vi "FPGA Main.vi"() -> ()   [LabVIEW 2014]
uses:
  <vilib>/Platform/TimedLoop/XDataNode/timing_clust.ctl
  <vilib>/Platform/TimedLoop/XDataNode/nitl_modes.ctl
  <vilib>/Platform/TimedLoop/XDataNode/wakeup.ctl
  <vilib>/rvi/eio/common/nirviEmuClasses.ctl
  <vilib>/rvi/Emulation/niFpgaGetClockAttributes.vi
  <vilib>/rvi/Emulation/niFpgaSctlEmulationGetInTimedLoop.vi
  <vilib>/rvi/Emulation/niFpgaEmulationReportErrorSimple.vi
  FPGA/VIs/FPGA Globals.vi
  <vilib>/rvi/Emulation/niFpgaProcessEmulError.vi
  <vilib>/rvi/eio/common/nirviEmuTemplateMethod_errors.vi
  <vilib>/rvi/Emulation/niFpgaCriticalErrorInLSC.vi
  <vilib>/rvi/interface/RandomDataEmulation/niFpgaRandomDataHandleErrors.vi
  <vilib>/eio/EIONode/EIONode.xnode
  <vilib>/eio/EIOGrowableMethodNode/genericMethod/EIOGrowableMethodNode.xnode
  <vilib>/rvi/eio/nirviEIOMethodImplementation/nirviEIOMethodImplementation.xnode
  <vilib>/rvi/eio/nirviErrorMerge/nirviErrorMerge.xnode
  <vilib>/rvi/DataTransferAndStorage/Container/XNode/niFpgaContainer.xnode
  <vilib>/rvi/interface/RandomDataEmulation/nirviRandomDataFpgaReadWriteTemplate.vi
  <vilib>/Platform/TimedLoop/XDataNode/XDataNode.xnode
  <vilib>/Platform/TimedLoop/XDataNode/XDNodeRunTimeDep.lvlib
panel:
  out "ADC First  Sample Recieved":bool
  out "Interlock HB":bool
  out "Global Triggered":bool
  in  "ADC Mask":bool[](array[boolean])=[FALSE, FALSE, FALSE, FALSE, FALSE, FALSE, FALSE, FALSE, FALSE, FALSE, FALSE, FALSE, FALSE, FALSE, FALSE, FALSE]
  out "DIN":bool[](array[boolean])
  out "ADC Triggered":bool
  out "DIN Triggered":bool
  out "ADC Min Threshold Triggered":bool[](array[boolean])
  out "ADC Max Threshold Triggered":bool[](array[boolean])
  in  "ADC Threshold max value":sgl[](array[numeric])=[0.0, 0.0, 0.0, 0.0, 0.0, 0.0, 0.0, 0.0, 0.0, 0.0, 0.0, 0.0, 0.0, 0.0, 0.0, 0.0]
  in  "ADC Threshold min value":sgl[](array[numeric])=[0.0, 0.0, 0.0, 0.0, 0.0, 0.0, 0.0, 0.0, 0.0, 0.0, 0.0, 0.0, 0.0, 0.0, 0.0, 0.0]
  out "Current sample":sgl[](array[numeric])
  out "ADC Sampling Timeout":bool
  out "Different Channel Count":bool
  out "Actual Loop Period (ticks)":u32
  in  "Interlock on":bool
  in  "Number of Channels":i16
  out "Data Acq Running":bool
  in  "Data Acq Stop":bool
  in  "External trigger":bool
  in  "Number samples\nafter trigger":i32
  in  "DIN Mask":bool[](array[boolean])=[FALSE, FALSE, FALSE, FALSE, FALSE, FALSE, FALSE, FALSE]
  in  "Sample Period (uSec)":u32=10
  out "Overwrite":bool
  out "Sample Gated":bool
  out "Error":bool
  out "FPGA Error":errorcluster
  out "DMA FIFO Full":bool
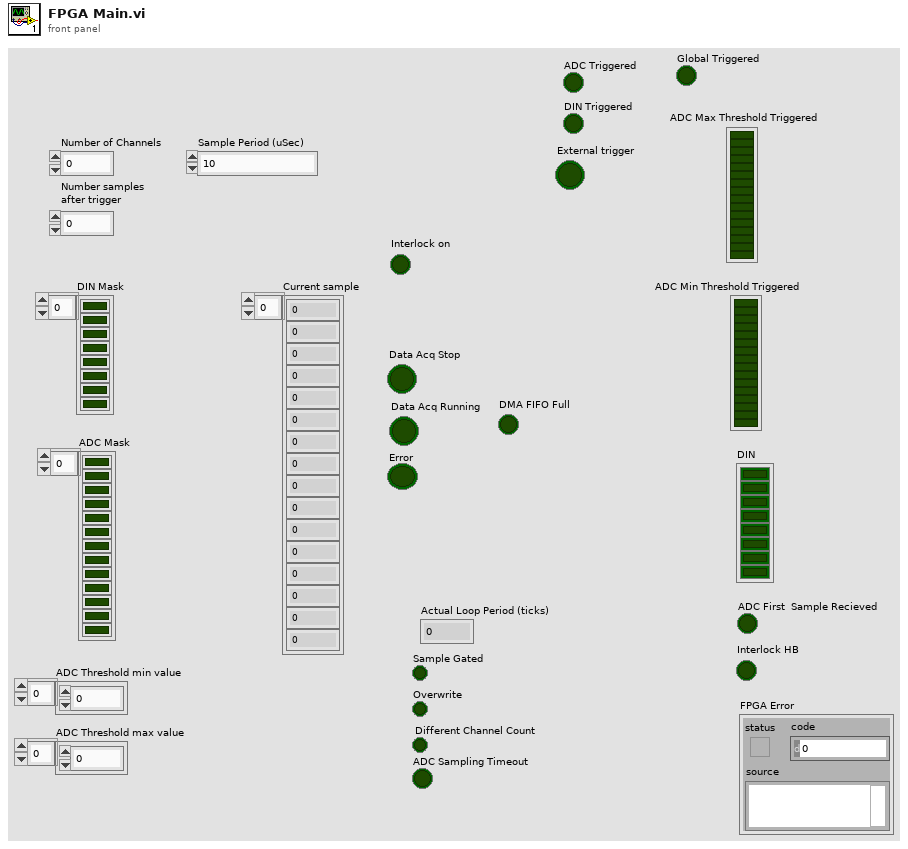
[diagram p1: front panel]
types:
  T1 = typedef "nirviEmuClasses.ctl" = enum16{"IO Read", "IO Write", "Method", "Property Read", "Property Write"}
  T2 = typedef "XDNodeRunTimeDep.lvlib/timing_clust.ctl" = cluster{"Expected End [f-1]":u64, "Actual End [f-1]":u64, "Finished Late? [f-1]":bool, "Expected End [i-1]":u64, "Actual End [i-1]":u64, "Finished Late? [i-1]":bool, "Expected Start [i]":u64, "Actual Start [i]":u64, "Expected Start [f]":u64, "Actual Start [f]":u64, "Source Name":string, "Structure Name":string, "Period":i64, "Deadline":i64, "Offset":i64, "Start":i64, "Priority":i32, "Timeout":i32, "Mode":T3, "Wakeup Reason":T4, "Error":errorcluster, "Source Type":string, "Secondary Source Type":string, "Global End Time":u64, "Global Start Time":u64, "Frame Duration":u64, "Iteration Duration":u64, "Assigned CPU":i32, "I/O Scan Engine Mode":u32}
  T3 = typedef "XDNodeRunTimeDep.lvlib/nitl_modes.ctl" = enum32{"No Change", "Process missed periods, maintain original phase", "Discard missed periods, maintain original phase", "Process missed periods, ignore original phase", "Discard missed periods, ignore original phase"}
  T4 = typedef "XDNodeRunTimeDep.lvlib/wakeup.ctl" = enum32{"Normal", "Aborted", "Asynchronous wakeup", "Timing source error", "Timed loop error", "Timeout"}
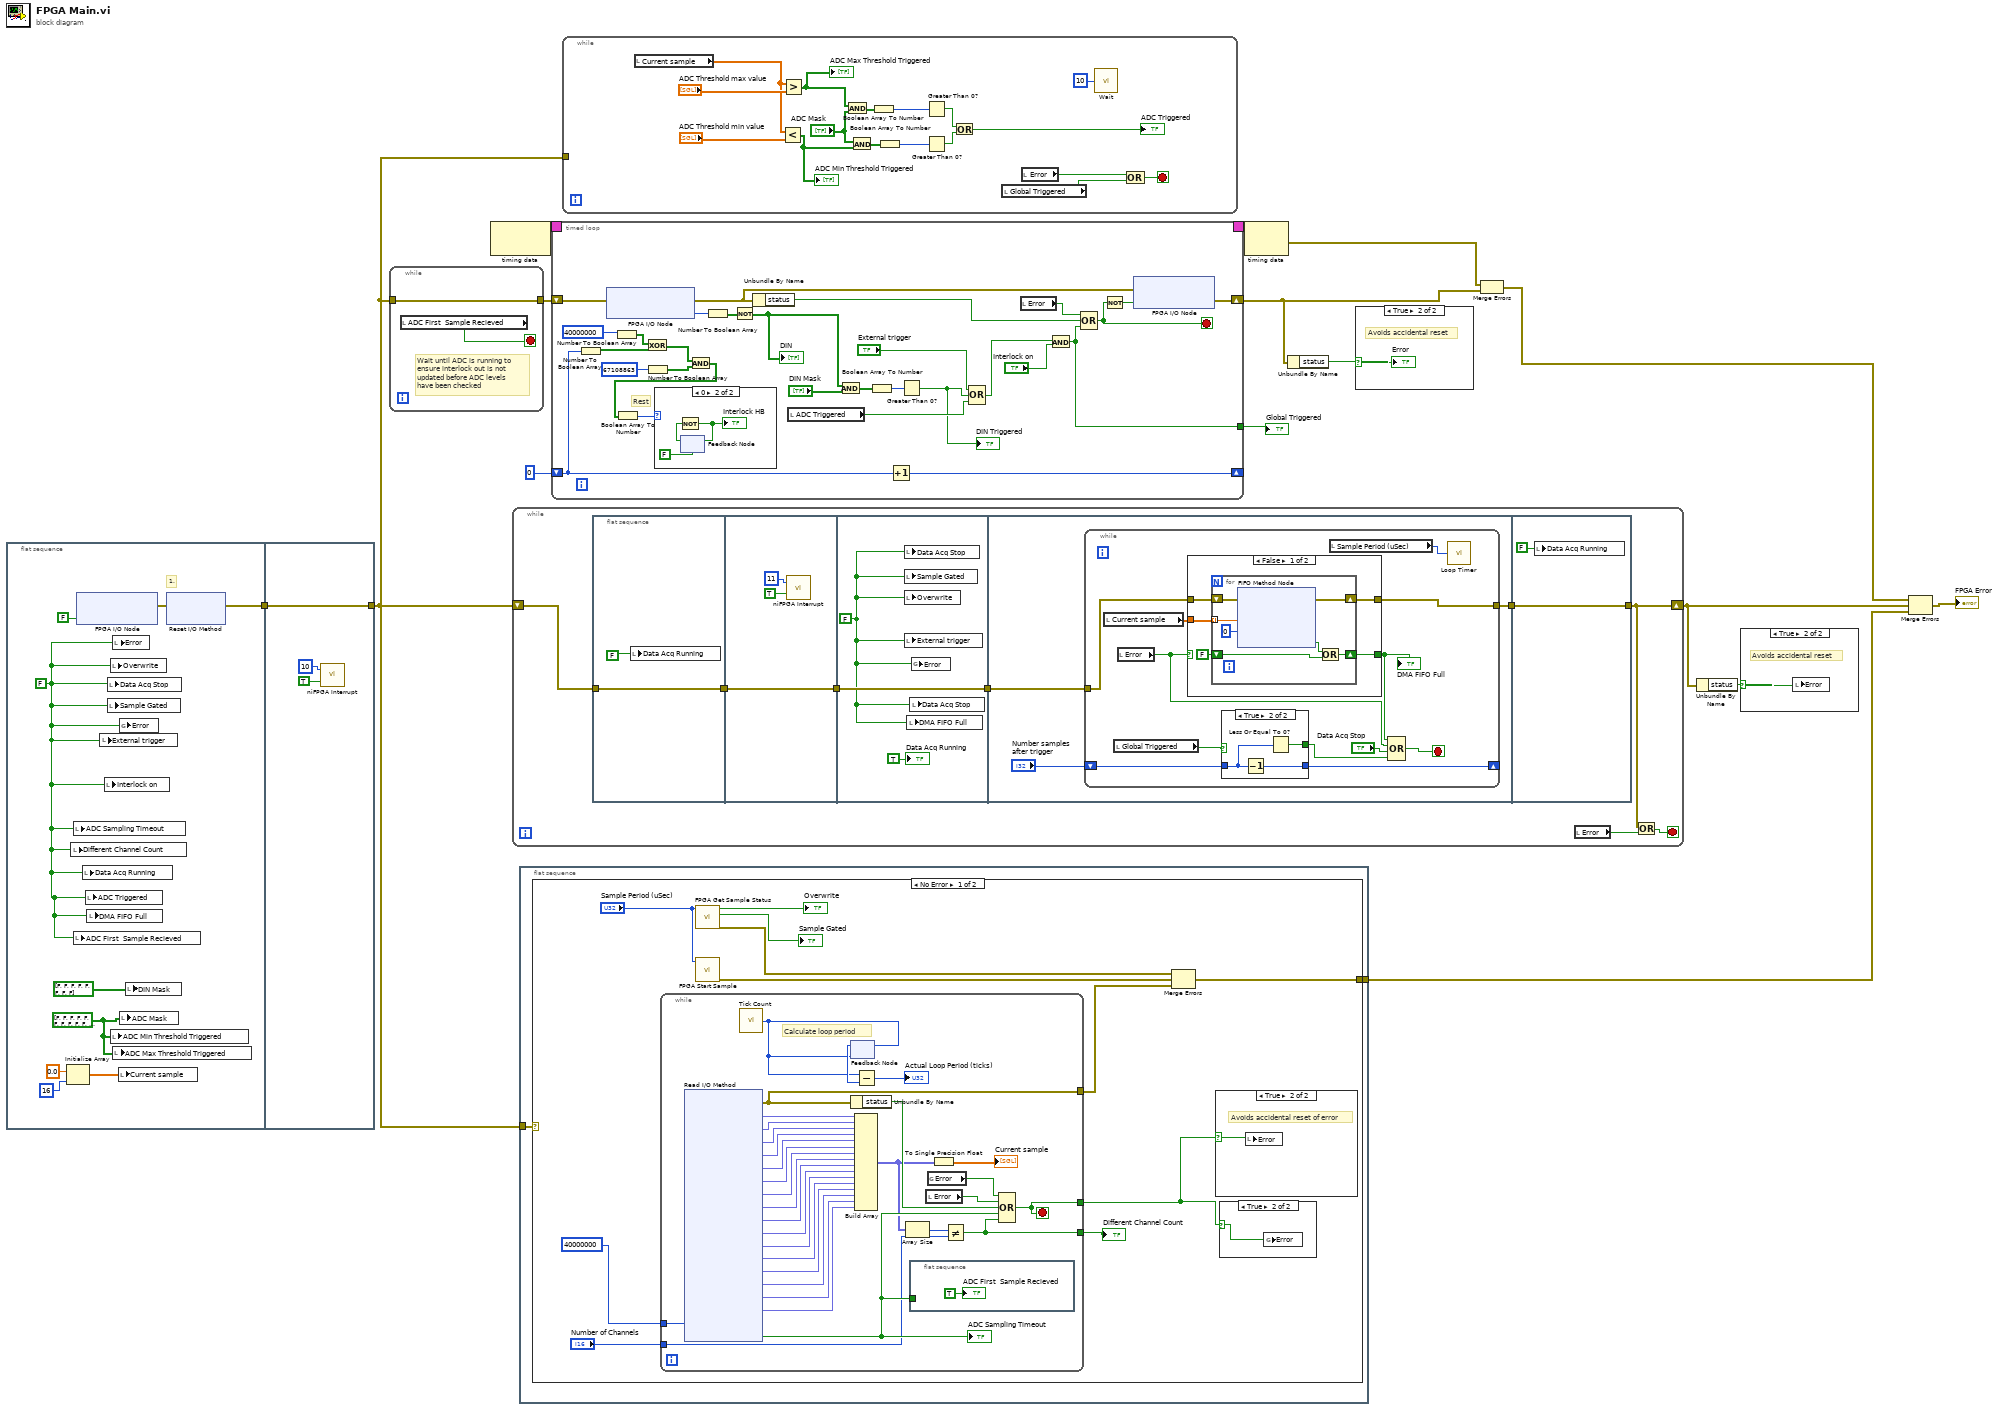
[diagram p0: block diagram]
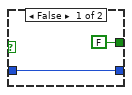
[diagram p8: hidden frame]
diagram:
  n1 = flat-sequence {
    tunnel: [w24] -> w11
    tunnel: [w71] -> w1
    tunnel: w11 -> [w71]
    frame #0 {
      w17 = bool[] [FALSE, FALSE, FALSE, FALSE, FALSE, FALSE, FALSE, FALSE, FALSE, FALSE, FALSE, FALSE, FALSE, FALSE, FALSE, FALSE] ("Mask")
      w16 = FALSE ("Stopped")
      # "1."
      n2 = Initialize Array(sgl 0.0 ("element"), 16 ("dimension size")) -> (w19:sgl[])
      n3 = local write "Different Channel Count"(w16) -> ()
      n4 = local write "ADC Sampling Timeout"(w16) -> ()
      n5 = local write "ADC First  Sample Recieved"(w16) -> ()
      n6 = xnode "FPGA I/O Node"("Mod1/DIO0"=FALSE) -> ("error out"=w23:errorcluster)  [unwired: 2 in, 1 out]
      n7 = local write "Data Acq Running"(w16) -> ()
      n8 = local write "ADC Triggered"(w16) -> ()
      n9 = local write "DMA FIFO Full"(w16) -> ()
      n10 = local write "External trigger"(w16) -> ()
      n11 = local write "Interlock on"(w16) -> ()
      n12 = local write "Data Acq Stop"(w16) -> ()
      n13 = local write "Sample Gated"(w16) -> ()
      n14 = local write "Overwrite"(w16) -> ()
      n15 = local write "ADC Min Threshold Triggered"(w17) -> ()
      n16 = local write "Error"(w16) -> ()
      n17 = local write "ADC Max Threshold Triggered"(w17) -> ()
      n18 = local write "Current sample"(w19) -> ()
      n19 = global write "FPGA Globals.vi" "Error"(w16) -> ()
      n20 = local write "ADC Mask"(w17) -> ()
      n21 = local write "DIN Mask"(bool[] [FALSE, FALSE, FALSE, FALSE, FALSE, FALSE, FALSE, FALSE] ("Mask")) -> ()
      n22 = xnode "Reset I/O Method"("error in"=w23) -> ("error out"=w24:errorcluster)  [unwired: 1 in, 1 out]
    }
    frame #1 {
      n23 = call <vilib>:"niFPGA Interrupt.vi"("Wait Until Cleared (F)"=TRUE ("Wait Until Cleared"), "IRQ Number (0)"=u8 10 ("IRQ Number")) -> ()  [unwired: 1 in]
    }
  }
  n24 = while {
    tunnel: [w73] -> w2
    tunnel: w1 -> [w73]
    stop <- w72 stop-if-true
    # "Wait until ADC is running to\nensure interlock out is not\nupdated before ADC levels\nhave been checked"
    n25 = local read "ADC First  Sample Recieved"() -> (w72:bool)
  }
  n26 = node-c288() -> (w13:T2)  [unwired: 1 in]
  n27 = while {
    shift-right: [w74] -> w4
    shift-left: w1 -> [w81]
    stop <- w75 stop-if-true
    n28 = flat-sequence {
      tunnel: w81 -> [w83]
      tunnel: [w83] -> w80
      tunnel: [w86] -> w79
      tunnel: w80 -> [w86]
      tunnel: w79 -> [w89]
      tunnel: [w89] -> w77
      tunnel: [w90] -> w76
      tunnel: w77 -> [w92]
      tunnel: w76 -> [w124]
      tunnel: [w124] -> w74
      frame #0 {
        n29 = local write "Data Acq Running"(FALSE ("DMA Running")) -> ()
      }
      frame #1 {
        n30 = call <vilib>:"niFPGA Interrupt.vi"("Wait Until Cleared (F)"=TRUE ("Wait Until Cleared"), "IRQ Number (0)"=u8 11 ("IRQ Number")) -> ()  [unwired: 1 in]
      }
      frame #2 {
        w87 = FALSE ("Stopped")
        n31 = local write "Data Acq Stop"(w87) -> ()
        n32 = local write "Sample Gated"(w87) -> ()
        n33 = local write "Overwrite"(w87) -> ()
        n34 = local write "External trigger"(w87) -> ()
        n35 = local write "DMA FIFO Full"(w87) -> ()
        n36 = local write "Data Acq Stop"(w87) -> ()
        n37 = global write "FPGA Globals.vi" "Error"(w87) -> ()
        "Data Acq Running" <- TRUE ("DMA Running")
      }
      frame #3 {
        n38 = while {
          tunnel: w92 -> [w104]
          tunnel: [w99] -> w90
          shift-right: [w98] -> _
          shift-left: "Number samples\nafter trigger" -> [w103]
          stop <- w102 stop-if-true
          n39 = local read "Current sample"() -> (w101:sgl[])
          n40 = local read "Global Triggered"() -> (w95:bool)
          n41 = local read "Error"() -> (w93:bool)
          n42 = case shown="False" w93 {
            selector: w93 -> [_ w122]
            tunnel: [w114 w123] -> w99
            tunnel: [w113 w122] -> w94
            tunnel: w104 -> [w112 w123]
            tunnel: w101 -> [w111 _]
            frame False {
              n43 = for {
                shift-right: [w120] -> w114
                shift-left: w112 -> [w121]
                shift-right: [w118] -> w113
                shift-left: FALSE -> [w117]
                tunnel: w111 -> [w115] mode=indexing
                n44 = xnode ("FIFO Method Node")("Element"=w115, "Timeout"=0, "error in (no error)"=w121) -> ("Timed Out?"=w119:bool, "error out"=w120:errorcluster)  [unwired: 1 in, 1 out]
                n45 = Or(x=w119, y=w117) -> (x .or. y?=w118:bool)
              }
            }
            frame True {
            }
          }
          "DMA FIFO Full" <- w94
          n46 = case shown="True" w95 {
            tunnel: [FALSE w108] -> w96
            tunnel: w103 -> [w105 w107]
            tunnel: [w105 w109] -> w98
            frame False {
            }
            frame True {
              n47 = Decrement(x=w107) -> (x-1=w109:i32)
              n48 = Less Or Equal To 0?(x=w107) -> (x <= 0?=w108:bool)
            }
          }
          n49 = local read "Sample Period (uSec)"() -> (w100:u32)
          n50 = Compound Arithmetic op=OR(w94, w93, "Data Acq Stop", w96) -> (w102:bool)
          n51 = call "Loop Timer"("Count(uSec)"=w100) -> ()  [unwired: 1 out]
        }
      }
      frame #4 {
        n52 = local write "Data Acq Running"(FALSE ("DMA Running")) -> ()
      }
    }
    n53 = local read "Error"() -> (w78:bool)
    n54 = Or(x=w74, y=w78) -> (x .or. y?=w75:bool)
  }
  n55 = flat-sequence {
    tunnel: w1 -> [w127]
    tunnel: [w126] -> w14
    frame #0 {
      n56 = case shown="No Error" w127 {
        selector: w127 -> [_ w785]
        tunnel: [w129 w785] -> w126
        frame No Error {
          n57 = while {
            tunnel: [w171] -> w130
            tunnel: 40000000 ("Timeout") -> [w165]
            tunnel: "Number of Channels" -> [w147]
            tunnel: [w146] -> w138
            tunnel: [w143] -> w128
            stop <- w143 stop-if-true
            # "Calculate loop period"
            n58 = xnode "Read I/O Method"("Timeout"=w165) -> ("error out"=w171:errorcluster, "Mod2/AI0"=w166:fxp<+/-,24,5>, "Mod2/AI1"=w164:fxp<+/-,24,5>, "Mod2/AI2"=w163:fxp<+/-,24,5>, "Mod2/AI3"=w162:fxp<+/-,24,5>, "Mod2/AI4"=w161:fxp<+/-,24,5>, "Mod2/AI5"=w160:fxp<+/-,24,5>, "Mod2/AI6"=w159:fxp<+/-,24,5>, "Mod2/AI7"=w158:fxp<+/-,24,5>, "Mod2/AI8"=w157:fxp<+/-,24,5>, "Mod2/AI9"=w156:fxp<+/-,24,5>, "Mod2/AI10"=w155:fxp<+/-,24,5>, "Mod2/AI11"=w154:fxp<+/-,24,5>, "Mod2/AI12"=w153:fxp<+/-,24,5>, "Mod2/AI13"=w152:fxp<+/-,24,5>, "Mod2/AI14"=w151:fxp<+/-,24,5>, "Mod2/AI15"=w150:fxp<+/-,24,5>, "Timed Out"=w149:bool)  [unwired: 17 in, 16 out]
            "ADC Sampling Timeout" <- w149
            n59 = call "Tick Count"() -> ("Tick Count(Ticks)"=w168:u32)
            n60 = feedback #1(w168) -> (w169:u32)
            n61 = feedback-in #1(w168) -> ()
            n62 = Unbundle By Name(w171) -> ("status"=w170:bool)
            n63 = Build Array(w166, w164, w163, w162, w161, w160, w159, w158, w157, w156, w155, w154, w153, w152, w151, w150) -> (w145:fxp<+/-,24,5>[])
            n64 = Subtract(x=w168, y=w169) -> (x-y=→"Actual Loop Period (ticks)":u32)
            n65 = Array Size(array=w145) -> (size(s)=w148:i32)
            n66 = flat-sequence {
              tunnel: w149 -> [_]
              frame #0 {
                "ADC First  Sample Recieved" <- TRUE ("ADC First  Sample recieved")
              }
            }
            n67 = local read "Error"() -> (w142:bool)
            n68 = global read "FPGA Globals.vi" "Error"() -> (w141:bool)
            n69 = To Single Precision Float(number=w145) -> (single precision float=→"Current sample":sgl[])
            n70 = Not Equal?(x=w148, y=w147) -> (x != y?=w146:bool)
            n71 = Compound Arithmetic op=OR(w141, w142, w170, w149, w146) -> (w143:bool)
          }
          "Different Channel Count" <- w138
          n72 = call "FPGA Get Sample Status.vi"("Sample Period (uSec)"="Sample Period (uSec)") -> ("error out"=w133:errorcluster, "Sample Gated"=→"Sample Gated":bool, "Overwrite"=→"Overwrite":bool)  [unwired: 8 in]
          n73 = call "FPGA Start Sample.vi"("Sample Period (uSec)"="Sample Period (uSec)") -> ("error out"=w134:errorcluster)  [unwired: 10 in]
          n74 = Merge Errors(w133, w134, w130) -> (w129:errorcluster)
          n75 = case shown="True" w128 {
            selector: w128 -> [_ w140]
            frame False {
            }
            frame True {
              # "Avoids accidental reset of error"
              n76 = local write "Error"(w140) -> ()
            }
          }
          n77 = case shown="True" w128 {
            selector: w128 -> [_ w139]
            frame False {
            }
            frame True {
              n78 = global write "FPGA Globals.vi" "Error"(w139) -> ()
            }
          }
        }
        frame Error {
        }
      }
    }
  }
  n79 = timed-loop {
    timing: w13 -> [_]
    timing-out: [_] -> w12
    shift-right: [w808] -> w7
    shift-left: w2 -> [w806]
    tunnel: [w799] -> w8
    shift-right: [w786] -> _
    shift-left: u64 0 -> [w787]
    stop <- w802 stop-if-true
    # "Rest"
    n80 = Number To Boolean Array(number=w787) -> (Boolean array=w793:bool[])
    n81 = xnode "FPGA I/O Node"("error in"=w806) -> ("error out"=w814:errorcluster, "Mod3/DIO7:0"=w809:u8)  [unwired: 1 in, 1 out]
    n82 = Number To Boolean Array(number=u64 40000000 ("y")) -> (Boolean array=w794:bool[])
    n83 = Exclusive Or(1:w793, 2:w794) -> (0:w791:bool[])
    n84 = Number To Boolean Array(number=u64 67108863 ("y")) -> (Boolean array=w790:bool[])
    n85 = And(x=w791, y=w790) -> (x .and. y?=w788:bool[])
    n86 = Boolean Array To Number(Boolean array=w788) -> (number=w789:u64)
    n87 = case shown="0" w789 {
      frame Default {
      }
      frame 0 {
        n88 = feedback #2(FALSE) -> (w817:bool)
        n89 = Not(x=w817) -> (.not. x?=w815:bool)
        "Interlock HB" <- w815
        n90 = feedback-in #2(w815) -> ()
      }
    }
    n91 = Number To Boolean Array(number=w809) -> (Boolean array=w811:bool[])
    n92 = Not(x=w811) -> (.not. x?=w798:bool[])
    "DIN" <- w798
    n93 = Unbundle By Name(w814) -> ("status"=w804:bool)
    n94 = local read "ADC Triggered"() -> (w805:bool)
    n95 = And(x=w798, y="DIN Mask") -> (x .and. y?=w813:bool[])
    n96 = Boolean Array To Number(Boolean array=w813) -> (number=w810:u8)
    n97 = Increment(x=w787) -> (x+1=w786:u64)
    n98 = Greater Than 0?(x=w810) -> (x > 0?=w800:bool)
    "DIN Triggered" <- w800
    n99 = Compound Arithmetic op=OR("External trigger", w800, w805) -> (w801:bool)
    n100 = local read "Error"() -> (w796:bool)
    n101 = And(x=w801, y="Interlock on") -> (x .and. y?=w799:bool)
    n102 = Compound Arithmetic op=OR(w796, w804, w799) -> (w802:bool)
    n103 = Not(x=w802) -> (.not. x?=w797:bool)
    n104 = xnode "FPGA I/O Node"("error in"=w814, "Mod1/DIO0"=w797) -> ("error out"=w808:errorcluster)  [unwired: 1 in, 1 out]
  }
  "Global Triggered" <- w8
  n105 = while {
    tunnel: w1 -> [_]
    stop <- w822 stop-if-true
    n106 = local read "Current sample"() -> (w828:sgl[])
    n107 = Less?(x=w828, y="ADC Threshold min value") -> (x < y?=w832:bool[])
    "ADC Min Threshold Triggered" <- w832
    n108 = Greater?(x=w828, y="ADC Threshold max value") -> (0:w826:bool[])
    "ADC Max Threshold Triggered" <- w826
    n109 = And(x=w826, y="ADC Mask") -> (x .and. y?=w827:bool[])
    n110 = And(x="ADC Mask", y=w832) -> (x .and. y?=w825:bool[])
    n111 = Boolean Array To Number(Boolean array=w827) -> (number=w833:u16)
    n112 = Boolean Array To Number(Boolean array=w825) -> (number=w834:u16)
    n113 = Greater Than 0?(x=w833) -> (x > 0?=w835:bool)
    n114 = Greater Than 0?(x=w834) -> (x > 0?=w836:bool)
    n115 = Or(x=w835, y=w836) -> (x .or. y?=→"ADC Triggered":bool)
    n116 = local read "Global Triggered"() -> (w820:bool)
    n117 = local read "Error"() -> (w823:bool)
    n118 = call "Wait"("Count(uSec)"=u32 10) -> ()  [unwired: 1 out]
    n119 = Compound Arithmetic op=OR(w823, w820) -> (w822:bool)
  }
  n120 = node-c288(w12) -> (w9:errorcluster)
  n121 = Unbundle By Name(w7) -> ("status"=w6:bool)
  n122 = case shown="True" w6 {
    selector: w6 -> [_ w837]
    frame False {
    }
    frame True {
      # "Avoids accidental reset"
      "Error" <- w837
    }
  }
  n123 = Merge Errors(w9, w7) -> (w10:errorcluster)
  n124 = Unbundle By Name(w4) -> ("status"=w5:bool)
  n125 = case shown="True" w5 {
    selector: w5 -> [_ w838]
    frame False {
    }
    frame True {
      # "Avoids accidental reset"
      n126 = local write "Error"(w838) -> ()
    }
  }
  n127 = Merge Errors(w10, w4, w14) -> (→"FPGA Error":errorcluster)
